vi "Init-FileHandler.vi"(5 "Formatter.lvclass":refnum<class "Formatter.lvclass">, 6 "Flush Timeout (5 s)":dbl=5.0, 7 "Filepath":path, 8 "error in":errorcluster, 9 "Level":T1, 10 "Name":string, 11 "FileHandler":refnum<class "RotateFileHandler.lvclass">) -> (0 "error out":errorcluster, 3 "FileHandler out":refnum<class "RotateFileHandler.lvclass">)   [LabVIEW 2024, in "RotateFileHandler.lvclass"]
doc: "Initiates a new FileHandler-object with a name, log-level and a filepath for the log-file.\nThe handler processes LogRecords only if the level of the handler is greater or equal to the level of the LogRecord.\n\n____\nHAMPEL SOFTWARE ENGINEERING v2.2.2 (2025-01-16 15:41)"
uses:
  RotateFileHandler.lvclass
  <vilib>/Hampel Software Engineering/HSE Logger/LogLevel.ctl
  <vilib>/Hampel Software Engineering/HSE Logger/Formatter/Formatter.lvclass
  RotateFileHandler.lvclass/RotateFileHandler.ctl
  <vilib>/Hampel Software Engineering/HSE Logger/hse-logger.lvlib
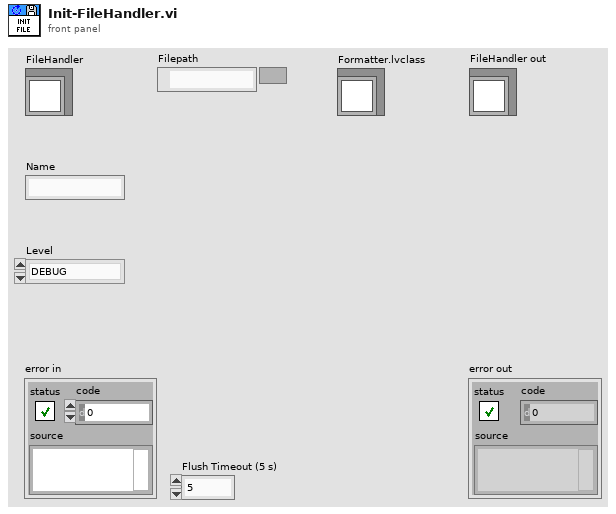
[diagram p1: front panel]
types:
  T1 = typedef "hse-logger.lvlib/LogLevel.ctl" = enum16{"DEBUG", "INFO", "WARNING", "ERROR", "CRITICAL"}
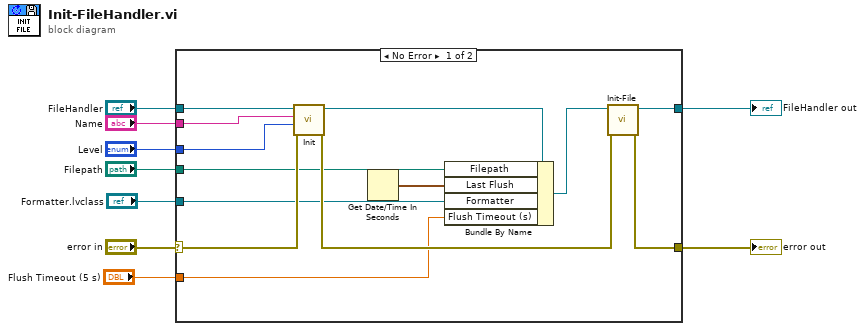
[diagram p0: block diagram]
diagram:
  n1 = case shown="No Error" "error in" {
    selector: "error in" -> [w21 w24]
    tunnel: [w12 w24] -> w8
    tunnel: [w10 w23] -> w7
    tunnel: "Name" -> [w20 _]
    tunnel: "Level" -> [w19 _]
    tunnel: "Filepath" -> [w13 _]
    tunnel: "FileHandler" -> [w18 w23]
    tunnel: "Flush Timeout (5 s)" -> [w15 _]
    tunnel: "Formatter.lvclass" -> [w14 _]
    frame No Error {
      n2 = call-dynamic "Init.vi"("error in"=w21, "Level"=w19, "Name"=w20, "Handler"=w18) -> ("error out"=w22:errorcluster, "Handler out"=w17:refnum<class "RotateFileHandler.lvclass">)  [unwired: 6 in]
      n3 = Get Date/Time In Seconds() -> (seconds since 1Jan1904=w16:timestamp)
      n4 = Bundle By Name(cluster=w17, "Filepath"=w13, "Last Flush"=w16, "Formatter"=w14, "Flush Timeout (s)"=w15) -> (w11:refnum<class "RotateFileHandler.lvclass">)
      n5 = call "Init-File.vi"("error in (no error)"=w22, "FileHandler in"=w11) -> ("error out"=w12:errorcluster, "FileHandler out"=w10:refnum<class "RotateFileHandler.lvclass">)  [unwired: 8 in]
    }
    frame Error {
    }
  }
  "error out" <- w8
  "FileHandler out" <- w7
